vi "HiLo2ErrorWarning.vi"(7 "value":dbl, 8 "lolo":dbl=-1e+100, 9 "lo":dbl=-1e+100, 10 "hi":dbl=1e+100, 11 "hihi":dbl=1e+100) -> (2 "warning":bool, 3 "error":bool)   [LabVIEW 2019]
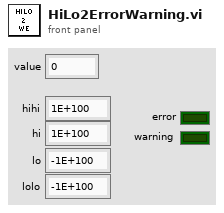
[diagram p1: front panel]
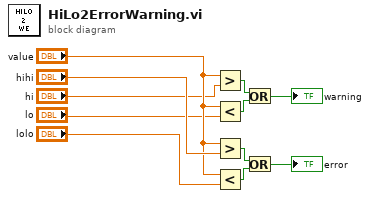
[diagram p0: block diagram]
diagram:
  n1 = Greater?(x="value", y="hi") -> (0:w7:bool)
  n2 = Less?(x="value", y="lo") -> (x < y?=w6:bool)
  n3 = Greater?(x="value", y="hihi") -> (0:w9:bool)
  n4 = Less?(x="value", y="lolo") -> (x < y?=w8:bool)
  n5 = Or(x=w7, y=w6) -> (x .or. y?=→"warning":bool)
  n6 = Or(x=w9, y=w8) -> (x .or. y?=→"error":bool)
